vi "SUM OF ‘n’ NATURAL NUMBERS USING WHILE.vi"() -> ()   [LabVIEW 2024]
panel:
  out "Output":dbl
  in  "Count":dbl
  in  "Constant":dbl
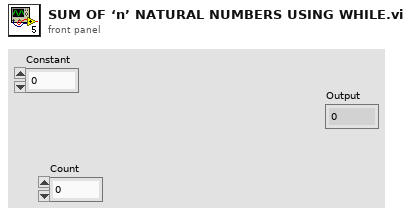
[diagram p1: front panel]
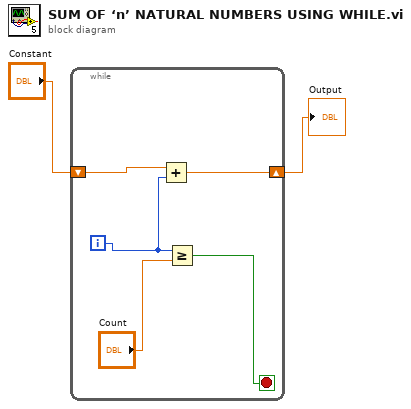
[diagram p0: block diagram]
diagram:
  n1 = while {
    shift-right: [w7] -> w2
    shift-left: "Constant" -> [w6]
    i -> [w4]
    stop <- w3 stop-if-true
    n2 = Add(x=w6, y=w4) -> (x+y=w7:dbl)
    n3 = Greater Or Equal?(x=w4, y="Count") -> (x >= y?=w3:bool)
  }
  "Output" <- w2
